vi "Error Cluster.Set Status.vi"(10 "status (T)":bool=TRUE, 11 "error in":errorcluster) -> (3 "error out":errorcluster)   [LabVIEW 2016, in "Memory Manager.lvlib" / "Static Error Handling.lvlib"]
doc: "Sets the error status of <b>error in</b>."
uses:
  Static Error Handling.lvlib
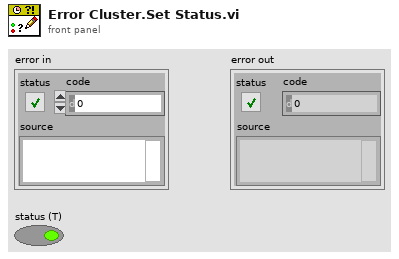
[diagram p1: front panel]
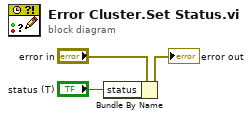
[diagram p0: block diagram]
diagram:
  n1 = Bundle By Name(cluster="error in", "status"="status (T)") -> (→"error out":errorcluster)
